vi "Redraw_data_raw_graph.vi"(8 "error in (no error)":errorcluster, 10 "Sel experiment":refnum<class "Experiment.lvclass">, 11 "Control-Client in":refnum<class "Control-Client.lvclass">) -> (0 "error out":errorcluster, 3 "Control-Client out":refnum<class "Control-Client.lvclass">)   [LabVIEW 2019, in "Control-Client.lvclass"]
uses:
  Control-Client.lvclass
  Experiments/Experiment.lvclass
  Control-Client.lvclass/Control-Client.ctl
  dependecies/average-2Darray-SD_int.vi
  dependecies/average-2Darray-SD_double.vi
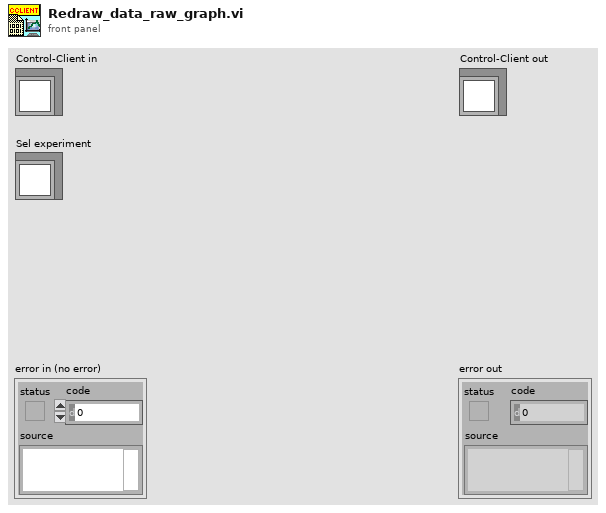
[diagram p1: front panel]
types:
  T1 = cluster{"Max Y pixel":i32, "Min Y pixel":i32, "Max X pixel":i32, "Min X pixel":i32}
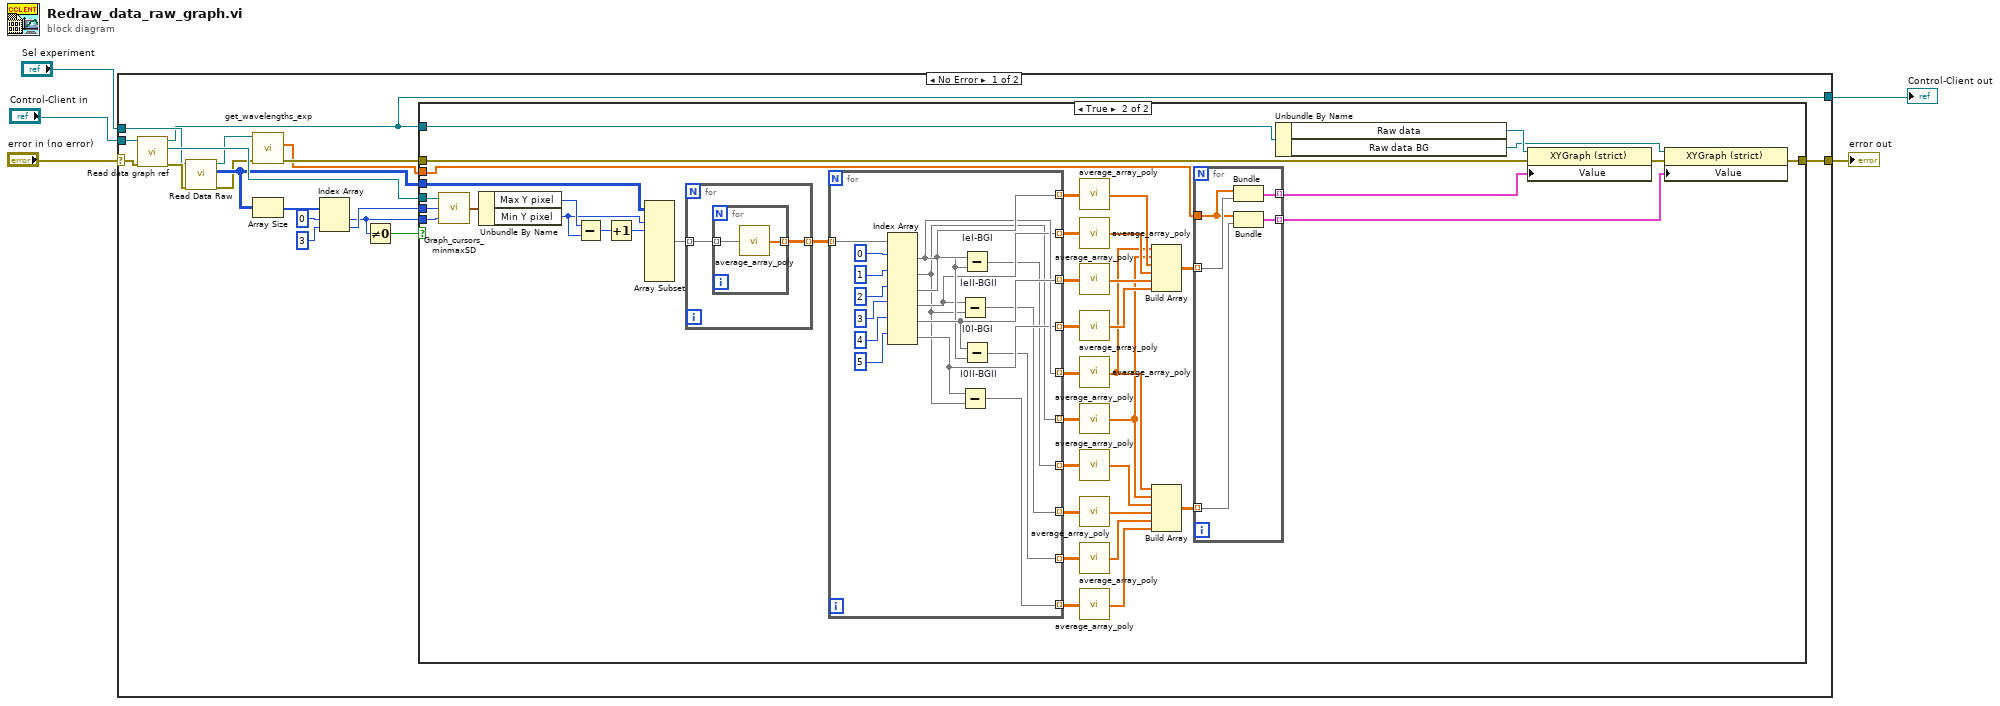
[diagram p0: block diagram]
diagram:
  n1 = case shown="No Error" "error in (no error)" {
    selector: "error in (no error)" -> [w23 w94]
    tunnel: [w8 w94] -> w4
    tunnel: [w14 w93] -> w2
    tunnel: "Control-Client in" -> [w21 w93]
    tunnel: "Sel experiment" -> [w19 _]
    frame No Error {
      n2 = call "Read data graph ref.vi"("error in (no error)"=w23, "Control-Client in"=w21) -> ("error out"=w20:errorcluster, "Exp data graph ref"=w22:refnum<vi>, "Control-Client out"=w14:refnum<class "Control-Client.lvclass">)  [unwired: 7 in]
      n3 = call-dynamic "Read Data Raw.vi"("error in (no error)"=w20, "Experiment in"=w19) -> ("error out"=w12:errorcluster, "Data Raw"=w13:i32[][][][], "Experiment out"=w11:refnum<class "Experiment.lvclass">)  [unwired: 7 in]
      n4 = call "get_wavelengths_exp.vi"("error in (no error)"=w12, "Experiment.lvclass in"=w11) -> ("error out"=w10:errorcluster, "wavelengths"=w9:dbl[])  [unwired: 7 in, 1 out]
      n5 = Array Size(array=w13) -> (size(s)=w18:i32[])
      n6 = Index Array(array=w18, index #1=0 ("index"), index #2=3 ("index")) -> (element #1=w7:i32, element #2=w15:i32)
      n7 = Not Equal To 0?(x=w7) -> (x != 0?=w6:bool)
      n8 = case shown="True" w6 {
        tunnel: w22 -> [_ w66]
        tunnel: w15 -> [_ w64]
        tunnel: w14 -> [_ w63]
        tunnel: w13 -> [_ w61]
        tunnel: w10 -> [w24 w54]
        tunnel: w9 -> [_ w42]
        tunnel: [w24 w38] -> w8
        tunnel: w7 -> [_ w25]
        frame False {
        }
        frame True {
          n9 = call "Graph_cursors_minmaxSD.vi"("Max Y pixel"=w25, "Max X pixel"=w64, "GRAPH EXPERIMENTAL DATA"=w66) -> ("max/min XY pixels"=w65:T1)
          n10 = Unbundle By Name(w65) -> ("Max Y pixel"=w62:i32, "Min Y pixel"=w60:i32)
          n11 = Subtract(x=w62, y=w60) -> (x-y=w59:i32)
          n12 = Increment(x=w59) -> (x+1=w58:i32)
          n13 = Array Subset(array=w61, index (dim 0)=w60, length (dim 0)=w58) -> (w56:i32[][][][])  [unwired: 6 in]
          n14 = for {
            tunnel: w56 -> [w90] mode=indexing
            tunnel: [w89] -> w55 mode=indexing
            n15 = for {
              tunnel: w90 -> [w92] mode=indexing
              tunnel: [w91] -> w89 mode=indexing
              n16 = call-poly "average_array_poly.vi"("2D array"=w92) -> ("out array"=w91:dbl[])
            }
          }
          n17 = for {
            tunnel: w55 -> [w88] mode=indexing
            tunnel: [w79] -> w53 mode=indexing
            tunnel: [w76] -> w52 mode=indexing
            tunnel: [w81] -> w51 mode=indexing
            tunnel: [w78] -> w50 mode=indexing
            tunnel: [w80] -> w49 mode=indexing
            tunnel: [w77] -> w48 mode=indexing
            tunnel: [w75] -> w35 mode=indexing
            tunnel: [w74] -> w33 mode=indexing
            tunnel: [w73] -> w31 mode=indexing
            tunnel: [w72] -> w28 mode=indexing
            n18 = Index Array(array=w88, index (row) #1=0 ("index (row)"), index (row) #2=1 ("index (row)"), index (row) #3=2 ("index (row)"), index (row) #4=3 ("index (row)"), index (row) #5=4 ("index (row)"), index (row) #6=5 ("index (row)")) -> (element #1=w79:dbl[], element #2=w76:dbl[], element #3=w81:dbl[], element #4=w78:dbl[], element #5=w80:dbl[], element #6=w77:dbl[])  [unwired: 6 in]
            n19 = Subtract "IeII-BGII"(x=w78, y=w76) -> (x-y=w74:dbl[])
            n20 = Subtract "I0II-BGII"(x=w77, y=w76) -> (x-y=w72:dbl[])
            n21 = Subtract "IeI-BGI"(x=w81, y=w79) -> (x-y=w75:dbl[])
            n22 = Subtract "I0I-BGI"(x=w80, y=w79) -> (x-y=w73:dbl[])
          }
          n23 = call-poly "average_array_poly.vi"("2D array"=w51) -> ("out array"=w47:dbl[])
          n24 = call-poly "average_array_poly.vi"("2D array"=w50) -> ("out array"=w46:dbl[])
          n25 = call-poly "average_array_poly.vi"("2D array"=w49) -> ("out array"=w45:dbl[])
          n26 = call-poly "average_array_poly.vi"("2D array"=w48) -> ("out array"=w44:dbl[])
          n27 = call-poly "average_array_poly.vi"("2D array"=w53) -> ("out array"=w37:dbl[])
          n28 = call-poly "average_array_poly.vi"("2D array"=w52) -> ("out array"=w36:dbl[])
          n29 = call-poly "average_array_poly.vi"("2D array"=w35) -> ("out array"=w34:dbl[])
          n30 = call-poly "average_array_poly.vi"("2D array"=w33) -> ("out array"=w32:dbl[])
          n31 = call-poly "average_array_poly.vi"("2D array"=w31) -> ("out array"=w30:dbl[])
          n32 = call-poly "average_array_poly.vi"("2D array"=w28) -> ("out array"=w29:dbl[])
          n33 = Build Array(w37, w36, w47, w46, w45, w44) -> (w43:dbl[][])
          n34 = Build Array(w37, w36, w34, w32, w30, w29) -> (w27:dbl[][])
          n35 = for {
            tunnel: w43 -> [w71] mode=indexing
            tunnel: w42 -> [w69]
            tunnel: [w70] -> w41 mode=indexing
            tunnel: w27 -> [w68] mode=indexing
            tunnel: [w67] -> w26 mode=indexing
            n36 = Bundle("wavelengths"=w69, w71) -> (w70:cluster{"wavelengths":dbl[], dbl[]})  [unwired: 1 in]
            n37 = Bundle("wavelengths"=w69, w68) -> (w67:cluster{"wavelengths":dbl[], dbl[]})  [unwired: 1 in]
          }
          n38 = Unbundle By Name(w63) -> ("Raw data"=w57:refnum<vi>, "Raw data BG"=w39:refnum<vi>)
          n39 = property class="XYGraph (strict)"(reference=w57, error in=w54, "Value"=w41) -> (error out=w40:errorcluster)  [unwired: 1 out]
          n40 = property class="XYGraph (strict)"(reference=w39, error in=w40, "Value"=w26) -> (error out=w38:errorcluster)  [unwired: 1 out]
        }
      }
    }
    frame Error {
    }
  }
  "error out" <- w4
  "Control-Client out" <- w2
